vi "Get Config File Path.vi"(8 "error in (no error)":errorcluster, 10 "Sphere indicator":T1, 11 "Base Path":path) -> (0 "error out":errorcluster, 2 "Cal File Folder":path, 3 "XML File Path":path)   [LabVIEW 2013, in "AvaSpec.lvlib" / "AvaSpec Settings.lvlib"]
doc: "Get the path to the Settings XML file. This is done using the Application Directory function. For more information on how Application Directory calculates its path, right-click the function and choose Help."
uses:
  AvaSpec Settings.lvlib
  Acquisition/Sphere Indicator.ctl
  AvaSpec.lvlib
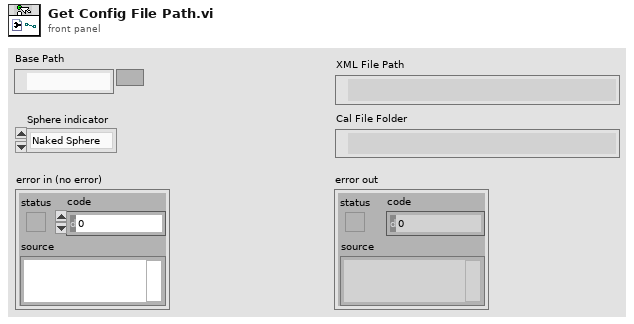
[diagram p1: front panel]
types:
  T1 = typedef "AvaSpec.lvlib/Sphere Indicator.ctl" = enum16{"Naked Sphere", "Insulated Sphere"}
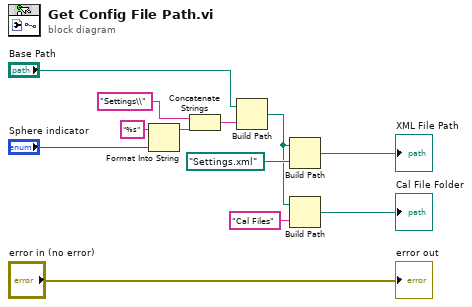
[diagram p0: block diagram]
diagram:
  n1 = Format Into String(format string="%s", "Sphere indicator") -> (resulting string=w8:string)  [unwired: 2 in, 1 out]
  n2 = Concatenate Strings("Settings\\" ("string"), w8) -> (w7:string)
  n3 = Build Path(base path="Base Path", name or relative path=w7) -> (appended path=w3:path)
  n4 = Build Path(base path=w3, name or relative path=path "Settings.xml" ("string")) -> (appended path=→"XML File Path":path)
  n5 = Build Path(base path=w3, name or relative path="Cal Files") -> (appended path=→"Cal File Folder":path)
  "error out" <- "error in (no error)"
